vi "EX5.vi"() -> ()   [LabVIEW 2018]
panel:
  in  "OK Button":bool
  in  "Operation":T1(ring)
  out "Result":dbl
  in  "B":dbl
  in  "A":dbl
  out "date string":string
  out "time string":string
  # "EX5 - TP0"
  # "Mekni Marwen 2ème Année Génie Electrique"
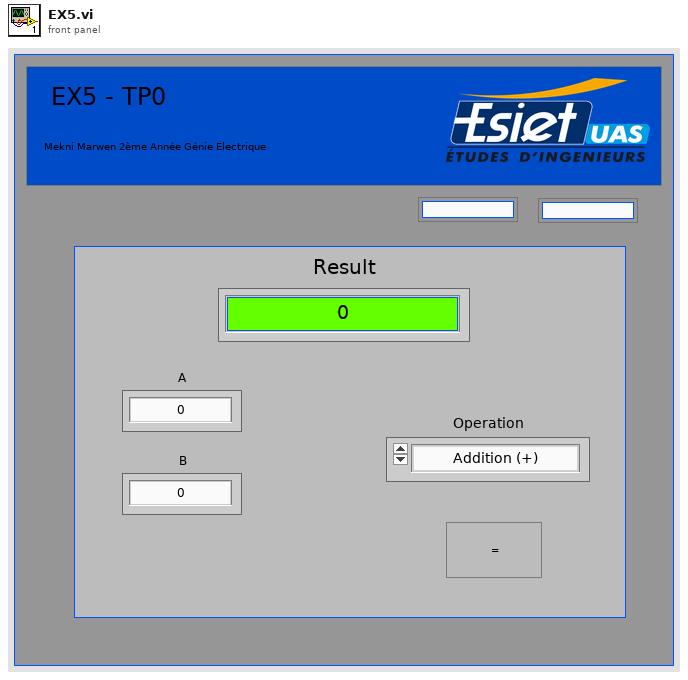
[diagram p1: front panel]
types:
  T1 = enum16{"Addition (+)", "Subtraction (-)", "Multiplication (×)", "Division (÷)"}
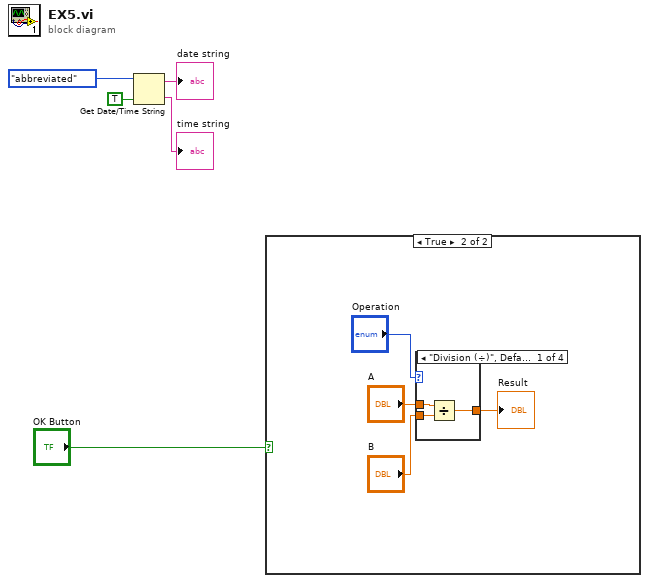
[diagram p0: block diagram]
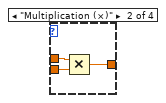
[diagram p3: hidden frame]
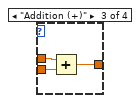
[diagram p4: hidden frame]
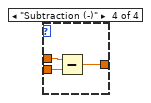
[diagram p5: hidden frame]
diagram:
  n1 = Get Date/Time String(date format (0)=enum16{"short", "long", "abbreviated"}."abbreviated", want seconds? (F)=TRUE) -> (date string=→"date string":string, time string=→"time string":string)  [unwired: 1 in]
  n2 = case shown="True" "OK Button" {
    frame False {
    }
    frame True {
      n3 = case shown="\"Division (÷)\", Default" "Operation" {
        tunnel: "A" -> [w12 w15 w17 w20]
        tunnel: "B" -> [w11 w14 w16 w19]
        tunnel: [w10 w13 w18 w21] -> w9
        frame "Division (÷)", Default {
          n4 = Divide(x=w12, y=w11) -> (x/y=w10:dbl)
        }
        frame "Multiplication (×)" {
          n5 = Multiply(x=w15, y=w14) -> (x*y=w13:dbl)
        }
        frame "Addition (+)" {
          n6 = Add(x=w17, y=w16) -> (x+y=w18:dbl)
        }
        frame "Subtraction (-)" {
          n7 = Subtract(x=w20, y=w19) -> (x-y=w21:dbl)
        }
      }
      "Result" <- w9
    }
  }
